vi "bgk_8001_reply.vi"(11 "unit reply":string caption="设备答复") -> (1 "reply parameter":string caption="答复参数", 2 "cmd code":string caption="指令代码", 3 "unit adress":string caption="设备地址", 4 "valid reply?":bool caption="合法答复?")   [LabVIEW 2015]
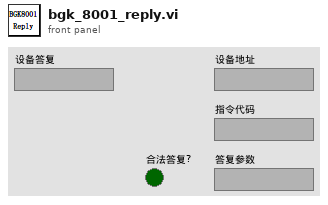
[diagram p1: front panel]
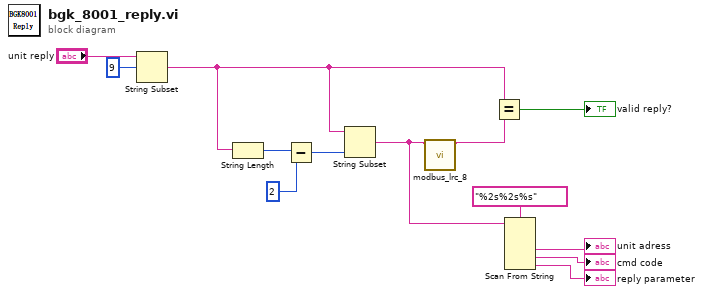
[diagram p0: block diagram]
diagram:
  n1 = String Subset(string="unit reply", offset (0)=9 ("偏移量(0)")) -> (substring=w13:string)  [unwired: 1 in]
  n2 = String Length(string=w13) -> (length=w10:i32)
  n3 = Subtract(x=w10, y=2) -> (x-y=w12:i32)
  n4 = String Subset(string=w13, length (rest)=w12) -> (substring=w2:string)  [unwired: 1 in]
  n5 = call "modbus_lrc_8.vi"("String"=w2) -> ("string & LRC-8"=w1:string)  [unwired: 8 in, 2 out]
  n6 = Equal?(x=w13, y=w1) -> (x = y?=→"valid reply?":bool)
  n7 = Scan From String(format string="%2s%2s%s" ("格式字符串"), input string=w2) -> (output 1=→"unit adress":string, output 2=→"cmd code":string, output 3=→"reply parameter":string)  [unwired: 5 in, 3 out]
